vi "RT-RNN.vi"(1 "Weights Cluster":T1, 2 "Input":dbl[](array[numeric])) -> (0 "Output":dbl[](array[numeric]))   [LabVIEW 2020]
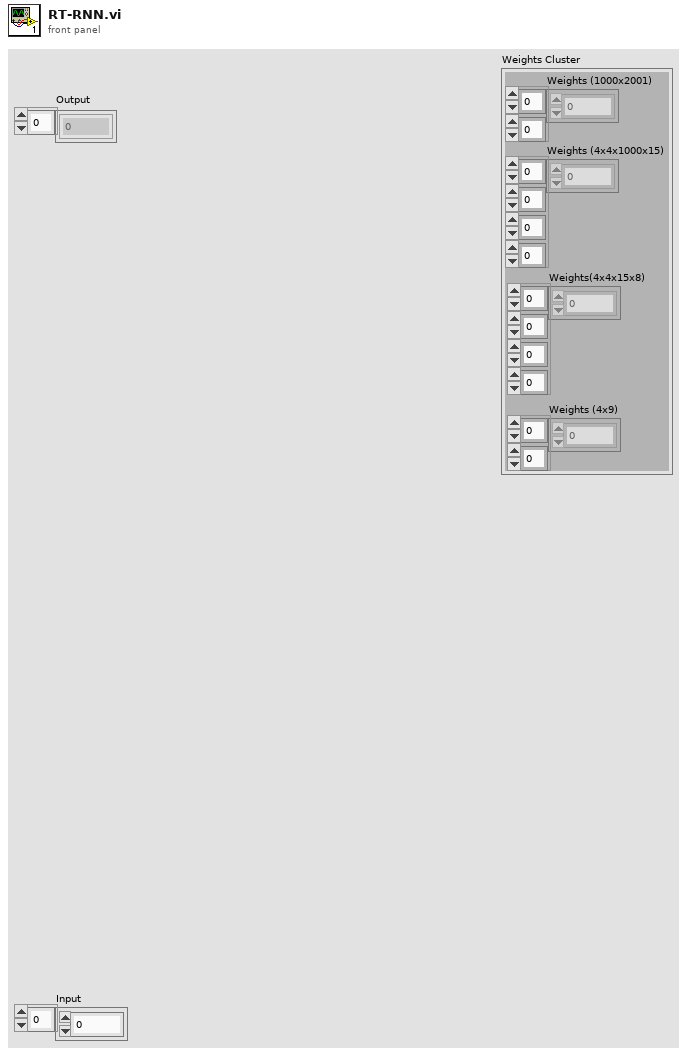
[diagram p1: front panel]
types:
  T1 = cluster{"Weights (1000x2001)":dbl[][], "Weights (4x4x1000x15)":dbl[][][][], "Weights(4x4x15x8)":dbl[][][][], "Weights (4x9)":dbl[][]}
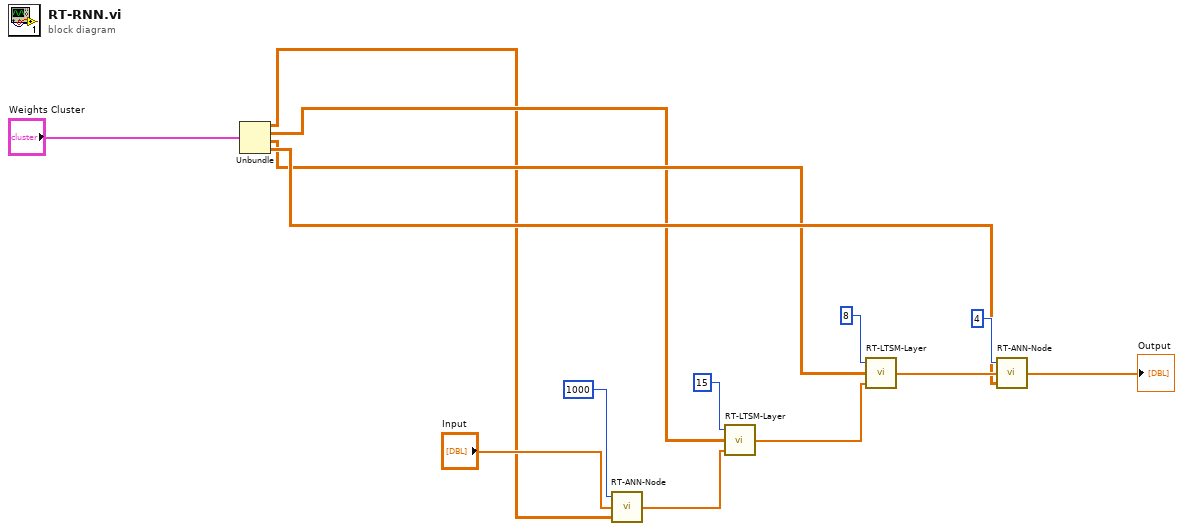
[diagram p0: block diagram]
diagram:
  n1 = Unbundle("Weights Cluster") -> ("Weights (1000x2001)"=w2:dbl[][], "Weights (4x4x1000x15)"=w3:dbl[][][][], "Weights(4x4x15x8)"=w4:dbl[][][][], "Weights (4x9)"=w5:dbl[][])
  n2 = call "RT-ANN-Node.vi"("Weights OutputSize x (InputSize + 1)"=w2, "Input"="Input", "Size of Output"=1000 ("Size")) -> ("Output"=w9:dbl[])
  n3 = call "RT-LTSM-Layer.vi"("Input Array"=w9, "Weights (4x4x1000x15)"=w3, "Layer Size"=15) -> ("Output Array"=w12:dbl[])
  n4 = call "RT-LTSM-Layer.vi"("Input Array"=w12, "Weights (4x4x1000x15)"=w4, "Layer Size"=8) -> ("Output Array"=w8:dbl[])
  n5 = call "RT-ANN-Node.vi"("Weights OutputSize x (InputSize + 1)"=w5, "Input"=w8, "Size of Output"=4) -> ("Output"=→"Output":dbl[])
